vi "Keithley2450 DC Pulses Blocks.vi"() -> ()   [LabVIEW 2020]
uses:
  <vilib>/Waveform/WDTOps.llb/WDT Append Waveforms DBL.vi
  <instrlib>/Keithley 2450/Public/Data/Read (Multiple Points).vi
  <vilib>/measure/NI_MAPro.lvlib
  <instrlib>/Keithley 2450/Keithley 2450.lvlib
  <instrlib>/Keithley 622x LV 2009/Keithley 622x.lvlib
panel:
  in  "Source Mode":enum16{"Voltage", "Current"}(ring)=enum."Current"
  in  "VISA resource name":refnum<visa-resource-name>
  in  "Compliance\nVoltage (V)":dbl=210.0
  out "Output Waveform":waveform(dbl)(graph)
  out "Total Time":dbl
  in  "Second Pulse\nTime (sec)":dbl
  in  "Second Pulse\nAmplitude (mU)":dbl
  in  "First Pulse\nTime (sec)":dbl
  in  "First Pulse\nAmplitude (mU)":dbl
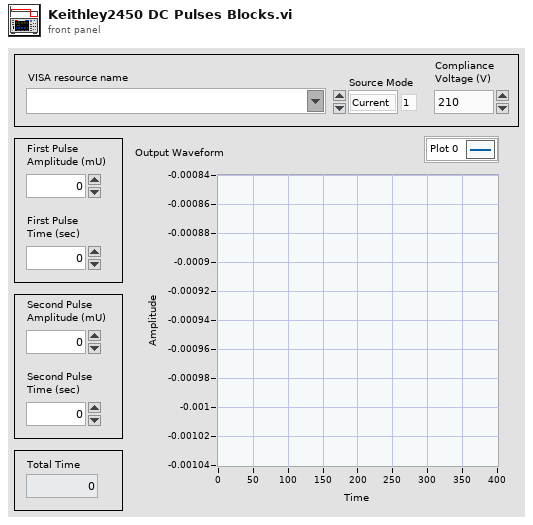
[diagram p1: front panel]
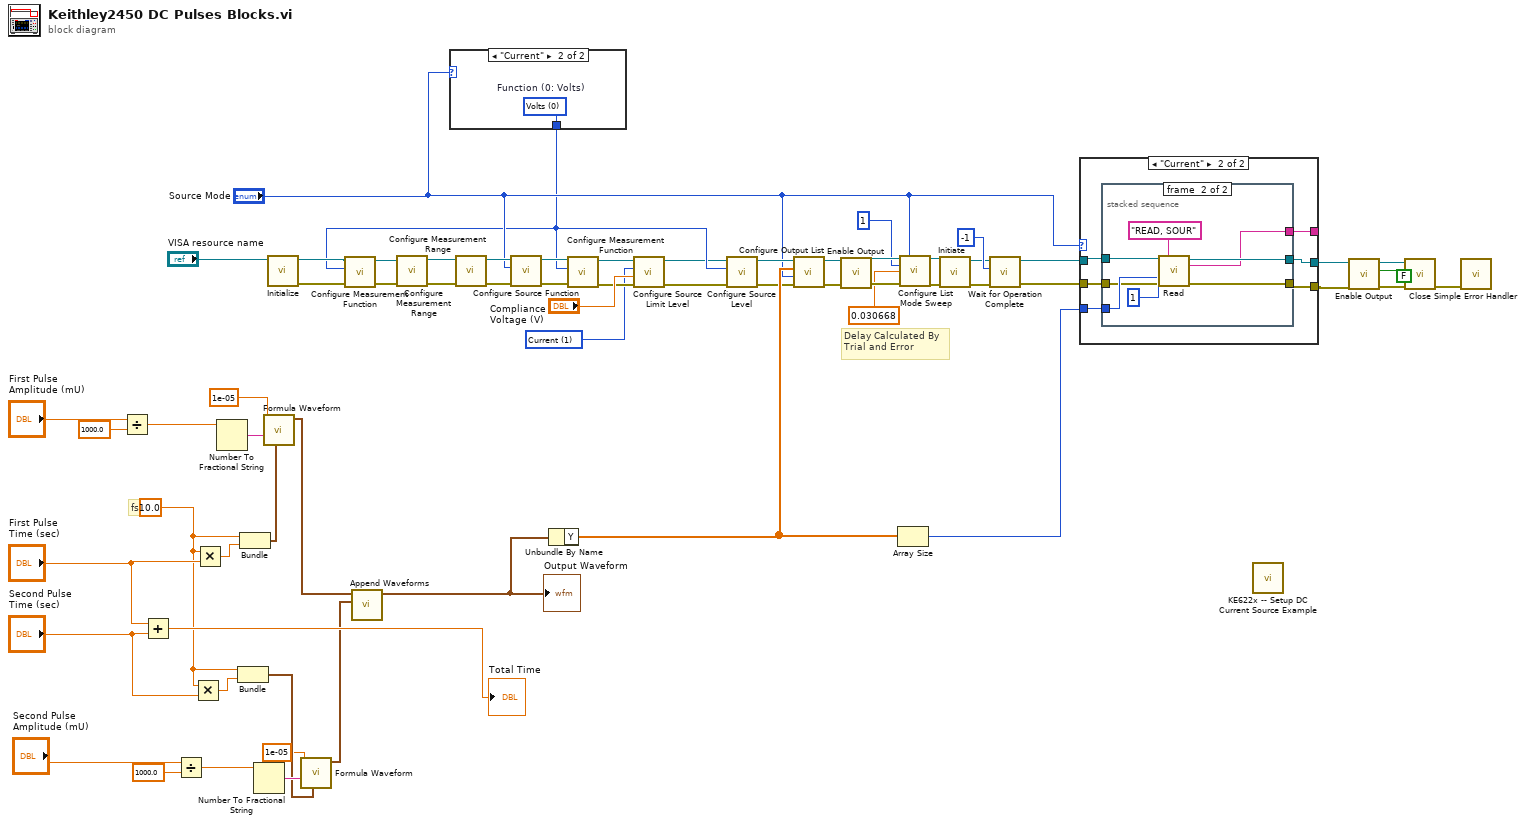
[diagram p0: block diagram]
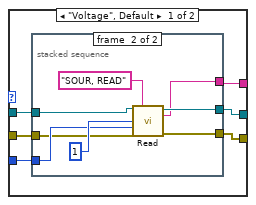
[diagram p2: hidden frame]
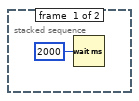
[diagram p3: hidden frame]
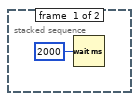
[diagram p4: hidden frame]
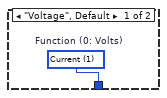
[diagram p5: hidden frame]
diagram:
  w12 = u16 1 items=["Volts", "Current"] ("Function (0: Volts)")
  w17 = 10.0
  # "Delay Calculated By\nTrial and Error"
  # "fs"
  n1 = Divide(x="First Pulse\nAmplitude (mU)", y=1000.0) -> (x/y=w6:dbl)
  n2 = Add(x="First Pulse\nTime (sec)", y="Second Pulse\nTime (sec)") -> (x+y=→"Total Time":dbl)
  n3 = Divide(x="Second Pulse\nAmplitude (mU)", y=1000.0) -> (x/y=w2:dbl)
  n4 = Multiply(x=w17, y="Second Pulse\nTime (sec)") -> (x*y=w62:dbl)
  n5 = Multiply(x=w17, y="First Pulse\nTime (sec)") -> (x*y=w63:dbl)
  n6 = Number To Fractional String(number=w6) -> (F-format string=w61:string)  [unwired: 3 in]
  n7 = Bundle(w17, w62) -> (w58:cluster{dbl, dbl})  [unwired: 1 in]
  n8 = Bundle(w17, w63) -> (w60:cluster{dbl, dbl})  [unwired: 1 in]
  n9 = Number To Fractional String(number=w2) -> (F-format string=w59:string)  [unwired: 3 in]
  n10 = call <vilib>:"Formula Waveform.vi"("sampling info"=w60, "formula"=w61, "frequency"=1e-05) -> ("signal out"=w57:waveform(dbl))  [unwired: 7 in, 1 out]
  n11 = call <instrlib>:"Initialize.vi"("VISA resource name"="VISA resource name") -> ("error out"=w41:errorcluster, "VISA resource name out"=w39:refnum<visa-resource-name>)  [unwired: 9 in]
  n12 = call <vilib>:"Formula Waveform.vi"("sampling info"=w58, "formula"=w59, "frequency"=1e-05) -> ("signal out"=w51:waveform(dbl))  [unwired: 7 in, 1 out]
  n13 = call-poly <vilib>:"Append Waveforms.vi"("waveform B"=w51, "waveform A"=w57) -> ("waveform out"=w50:waveform(dbl))  [unwired: 8 in, 1 out]
  "Output Waveform" <- w50
  n14 = case shown="\"Current\"" "Source Mode" {
    tunnel: [w64 w65] -> w13
    frame "Voltage", Default {
      w64 = u16 1 items=["Volts", "Current", "Resistance"]  # Function (0: Volts)
    }
    frame "Current" {
      w65 = u16 0 items=["Volts", "Current", "Resistance"]  # Function (0: Volts)
    }
  }
  n15 = call <instrlib>:"Configure Measurement Function.vi"("error in (no error)"=w41, "Function (0: Volts)"=w13, "VISA resource name"=w39) -> ("error out"=w40:errorcluster, "VISA resource name out"=w38:refnum<visa-resource-name>)  [unwired: 7 in]
  n16 = call <instrlib>:"Configure Measurement Range.vi"("error in (no error)"=w40, "VISA resource name"=w38) -> ("error out"=w49:errorcluster, "VISA resource name out"=w48:refnum<visa-resource-name>)  [unwired: 8 in]
  n17 = call <instrlib>:"Configure Measurement Range.vi"("error in (no error)"=w49, "VISA resource name"=w48) -> ("error out"=w37:errorcluster, "VISA resource name out"=w36:refnum<visa-resource-name>)  [unwired: 8 in]
  n18 = call <instrlib>:"Configure Source Function.vi"("error in (no error)"=w37, "Function (0: Volts)"="Source Mode", "VISA resource name"=w36) -> ("error out"=w24:errorcluster, "VISA resource name out"=w27:refnum<visa-resource-name>)  [unwired: 7 in]
  n19 = Unbundle By Name(w50) -> ("Y"=w22:dbl[])
  n20 = call <instrlib>:"Configure Measurement Function.vi"("error in (no error)"=w24, "Function (0: Volts)"=w13, "VISA resource name"=w27) -> ("error out"=w25:errorcluster, "VISA resource name out"=w26:refnum<visa-resource-name>)  [unwired: 7 in]
  n21 = call <instrlib>:"Configure Source Limit Level.vi"("error in (no error)"=w25, "Source Limit (1.0)"="Compliance\nVoltage (V)", "Function (0: Volts)"=w12, "VISA resource name"=w26) -> ("error out"=w8:errorcluster, "VISA resource name out"=w9:refnum<visa-resource-name>)  [unwired: 6 in]
  n22 = call <instrlib>:"Configure Source Level.vi"("error in (no error)"=w8, "Function (0: Volts)"=w13, "VISA resource name"=w9) -> ("error out"=w18:errorcluster, "VISA resource name out"=w19:refnum<visa-resource-name>)  [unwired: 7 in]
  n23 = call <instrlib>:"Configure Output List.vi"("error in (no error)"=w18, "Source Mode  (0: Voltage)"="Source Mode", "Output List"=w22, "VISA resource name"=w19) -> ("error out"=w44:errorcluster, "VISA resource name out"=w45:refnum<visa-resource-name>)  [unwired: 6 in]
  n24 = call <instrlib>:"Enable Output.vi"("error in (no error)"=w44, "VISA resource name"=w45) -> ("error out"=w35:errorcluster, "VISA resource name out"=w34:refnum<visa-resource-name>)  [unwired: 8 in]
  n25 = Array Size(array=w22) -> (size(s)=w21:i32)
  n26 = call <instrlib>:"Configure List Mode Sweep.vi"("VISA resource name"=w34, "Source Mode  (0: Voltage)"="Source Mode", "Start Index"=u32 1, "Delay (0)"=0.030668, "error in (no error)"=w35) -> ("VISA resource name out"=w32:refnum<visa-resource-name>, "error out"=w31:errorcluster)  [unwired: 9 in]
  n27 = call <instrlib>:"Initiate.vi"("error in (no error)"=w31, "VISA resource name"=w32) -> ("error out"=w29:errorcluster, "VISA resource name out"=w7:refnum<visa-resource-name>)  [unwired: 8 in]
  n28 = call <instrlib>:"Wait for Operation Complete.vi"("error in (no error)"=w29, "Timeout (10000 ms)"=-1, "VISA resource name"=w7) -> ("error out"=w23:errorcluster, "VISA resource name out"=w15:refnum<visa-resource-name>)  [unwired: 7 in]
  n29 = case shown="\"Current\"" "Source Mode" {
    tunnel: [w71 w85] -> w11
    tunnel: [w70 w84] -> w10
    tunnel: w21 -> [w69 w86]
    tunnel: [w68 w83] -> _
    tunnel: w23 -> [w67 w82]
    tunnel: w15 -> [w66 w81]
    frame "Voltage", Default {
      n30 = stacked-sequence {
        tunnel: [_ w80] -> w71
        tunnel: [_ w79] -> w70
        tunnel: [_ w77] -> w68
        tunnel: w69 -> [_ w75]
        tunnel: w67 -> [_ w74]
        tunnel: w66 -> [_ w73]
        frame #0 {
          n31 = Wait (ms)(milliseconds to wait=u32 2000) -> ()  [unwired: 1 out]
        }
        frame #1 {
          n32 = call-poly <instrlib>:"Read.vi"("VISA resource name"=w73, "Buffer Elements"="SOUR, READ", "Start Index (1)"=1, "End Index (1)"=w75, "error in (no error)"=w74) -> ("VISA resource name out"=w80:refnum<visa-resource-name>, "Data out"=w77:string, "error out"=w79:errorcluster)  [unwired: 8 in]
        }
      }
    }
    frame "Current" {
      n33 = stacked-sequence {
        tunnel: [_ w95] -> w85
        tunnel: [_ w94] -> w84
        tunnel: [_ w92] -> w83
        tunnel: w86 -> [_ w90]
        tunnel: w82 -> [_ w89]
        tunnel: w81 -> [_ w88]
        frame #0 {
          n34 = Wait (ms)(milliseconds to wait=u32 2000) -> ()  [unwired: 1 out]
        }
        frame #1 {
          n35 = call-poly <instrlib>:"Read.vi"("VISA resource name"=w88, "Buffer Elements"="READ, SOUR", "Start Index (1)"=1, "End Index (1)"=w90, "error in (no error)"=w89) -> ("VISA resource name out"=w95:refnum<visa-resource-name>, "Data out"=w92:string, "error out"=w94:errorcluster)  [unwired: 8 in]
        }
      }
    }
  }
  n36 = call <instrlib>:"KE622x -- Setup DC Current Source Example.vi"() -> ()  [unwired: 1 in]
  n37 = call <instrlib>:"Enable Output.vi"("error in (no error)"=w10, "Enable Output (T: Enable)"=FALSE, "VISA resource name"=w11) -> ("error out"=w43:errorcluster, "VISA resource name out"=w42:refnum<visa-resource-name>)  [unwired: 7 in]
  n38 = call <instrlib>:"Close.vi"("error in (no error)"=w43, "VISA resource name"=w42) -> ("error out"=w46:errorcluster)  [unwired: 9 in]
  n39 = call <vilib>:"Simple Error Handler.vi"("error in (no error)"=w46) -> ()  [unwired: 4 in, 5 out]
